vi "Avantes - AVS_StopMeasure.vi"(8 "error in (no error)":errorcluster, 11 "Cluster in":T1) -> (0 "error out":errorcluster, 3 "Cluster out":T1)   [LabVIEW 2013, in "Avantes Spectrometer Functions.lvlib"]
uses:
  Avantes Spectrometer Functions.lvlib
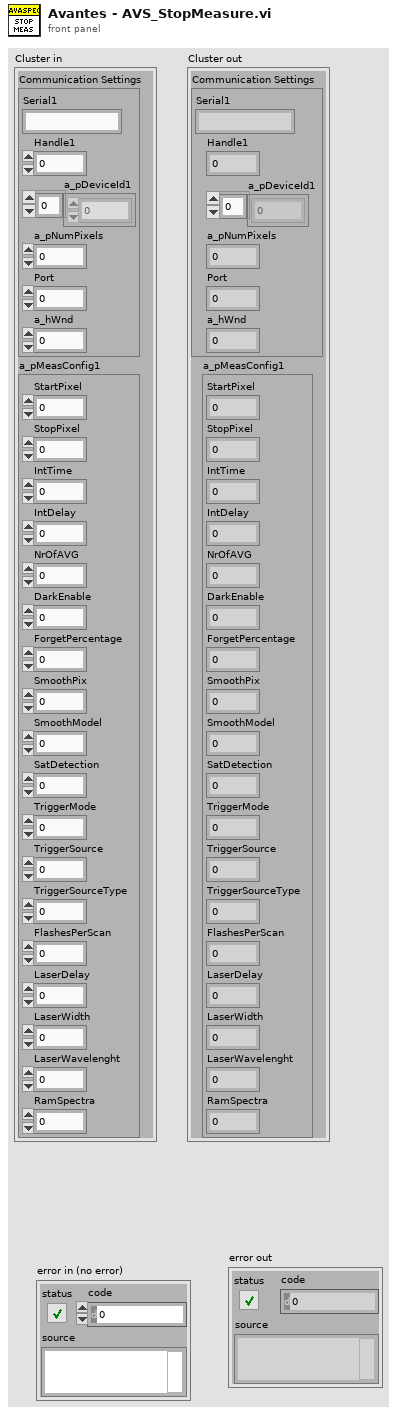
[diagram p1: front panel]
types:
  T1 = cluster{"Communication Settings":cluster{"Serial1":string, "Handle1":i32, "a_pDeviceId1":u8[], "a_pNumPixels":u16, "Port":i32, "a_hWnd":i32}, "a_pMeasConfig1":cluster{"StartPixel":u16, "StopPixel":u16, "IntTime":sgl, "IntDelay":u32, "NrOfAVG":u32, "DarkEnable":u8, "ForgetPercentage":u8, "SmoothPix":u16, "SmoothModel":u8, "SatDetection":u8, "TriggerMode":u8, "TriggerSource":u8, "TriggerSourceType":u8, "FlashesPerScan":u16, "LaserDelay":u32, "LaserWidth":u32, "LaserWavelenght":sgl, "RamSpectra":u16}}
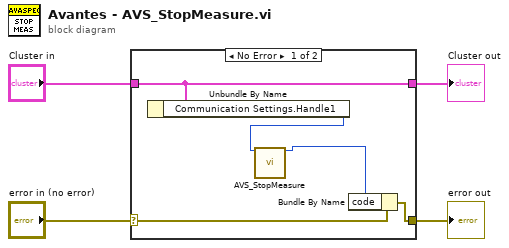
[diagram p0: block diagram]
diagram:
  n1 = case shown="No Error" "error in (no error)" {
    selector: "error in (no error)" -> [w8 w11]
    tunnel: [w9 w10] -> w4
    tunnel: "Cluster in" -> [w9 w10]
    tunnel: [w7 w11] -> w1
    frame No Error {
      n2 = Unbundle By Name(w9) -> ("Communication Settings.Handle1"=w6:i32)
      n3 = call "AVS_StopMeasure.vi"("a_hDevice"=w6) -> ("Output Value"=w5:i32)  [unwired: 14 in]
      n4 = Bundle By Name(cluster=w8, "code"=w5) -> (w7:errorcluster)
    }
    frame Error {
    }
  }
  "Cluster out" <- w4
  "error out" <- w1
